vi "ASCOM61_test.vi"() -> ()   [LabVIEW 2010]
panel:
  out "error out":errorcluster
  out "Declination":dbl
  out "RightAscension":dbl
  in  "Quit":bool
  out "DriverInfo":string
  in  "reference":refnum<k7>
  out "Connected":bool
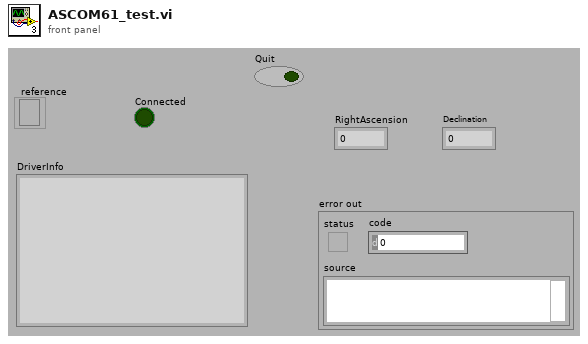
[diagram p1: front panel]
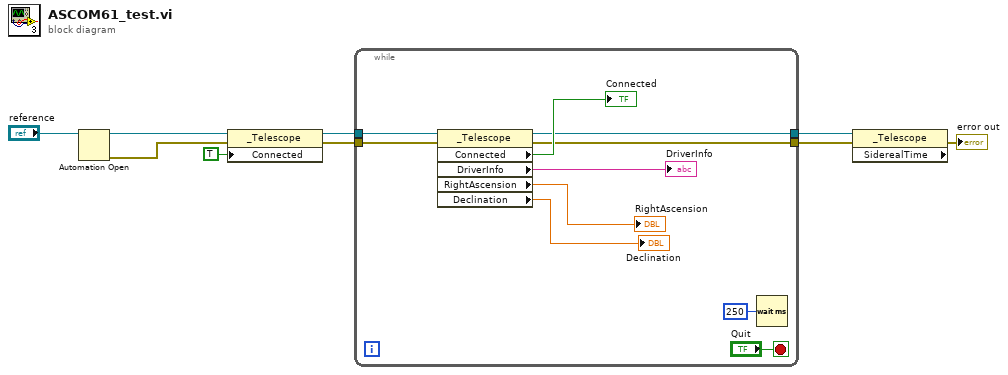
[diagram p0: block diagram]
diagram:
  n1 = Automation Open(Automation Refnum="reference") -> (Automation Refnum=w1:refnum<k7>, error out=w2:errorcluster)  [unwired: 3 in]
  n2 = property class="_Telescope"(reference=w1, error in=w2, "Connected"=TRUE) -> (reference out=w4:refnum<k7>, error out=w3:errorcluster)
  n3 = while {
    tunnel: w4 -> [w18]
    tunnel: [w14] -> w8
    tunnel: [w11] -> w7
    tunnel: w3 -> [w10]
    stop <- "Quit" stop-if-true
    n4 = property class="_Telescope"(reference=w18, error in=w10) -> (reference out=w14:refnum<k7>, error out=w11:errorcluster, "Connected"=→"Connected":bool, "DriverInfo"=→"DriverInfo":string, "RightAscension"=→"RightAscension":dbl, "Declination"=→"Declination":dbl)
    n5 = Wait (ms)(milliseconds to wait=u32 250) -> ()  [unwired: 1 out]
  }
  n6 = property class="_Telescope" props=["SiderealTime"](reference=w8, error in=w7) -> (error out=→"error out":errorcluster)  [unwired: 2 out]
